vi "Close Instrument Sessions.vi"(0 "Vector Path Group in":refnum<class "Vector 18GHz Path Group.lvclass">, 11 "error in (no error)":errorcluster) -> (4 "Vector Path Group out":refnum<class "Vector 18GHz Path Group.lvclass">, 15 "error out":errorcluster)   [LabVIEW 2023, in "RFFixtureCharact.RFPM.lvlib" / "Vector 18GHz Path Group.lvclass"]
uses:
  Vector 18GHz Path Group.lvclass
  Vector 18GHz Path Group.lvclass/Vector 18GHz Path Group.ctl
  Public/Base Classes/Vector/Vector Abstract Path Group/Vector Abstract Path Group.lvclass
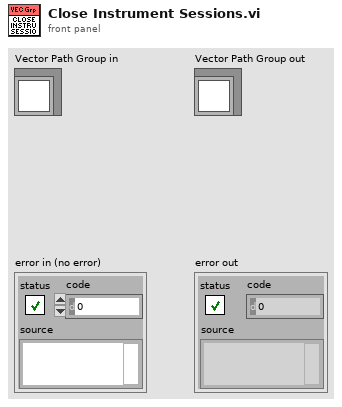
[diagram p1: front panel]
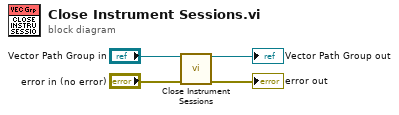
[diagram p0: block diagram]
diagram:
  n1 = call-parent "Close Instrument Sessions.vi"("Vector Abstract Path Group in"="Vector Path Group in", "error in (no error)"="error in (no error)") -> ("Vector Abstract Path Group out"=→"Vector Path Group out":refnum<class "Vector 18GHz Path Group.lvclass">, "error out"=→"error out":errorcluster)  [unwired: 12 in]
